vi "D3X86 GPIB Error check.vi"(1 "GPIB Error":i16, 2 "Status":bool[](array[boolean])) -> (0 "Error":bool)   [LabVIEW 2017]
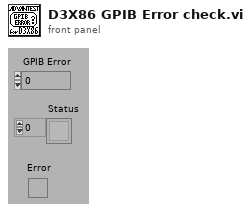
[diagram p1: front panel]
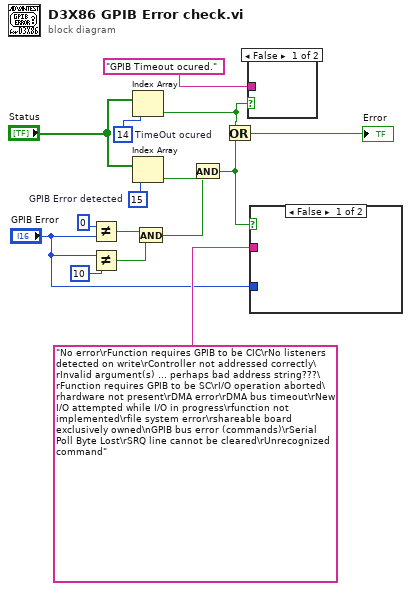
[diagram p0: block diagram]
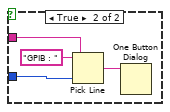
[diagram p2: hidden frame]
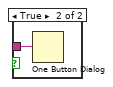
[diagram p3: hidden frame]
diagram:
  w14 = 14  # TimeOut ocured
  w15 = 15  # GPIB Error detected
  n1 = Not Equal?(x=u16 0, y="GPIB Error") -> (x != y?=w2:bool)
  n2 = Not Equal?(x="GPIB Error", y=10) -> (x != y?=w1:bool)
  n3 = Index Array(array="Status", index=w14) -> (element=w9:bool)
  n4 = Index Array(array="Status", index=w15) -> (element=w13:bool)
  n5 = And(x=w2, y=w1) -> (x .and. y?=w3:bool)
  n6 = And(x=w13, y=w3) -> (x .and. y?=w8:bool)
  n7 = Or(x=w9, y=w8) -> (x .or. y?=→"Error":bool)
  n8 = case shown="False" w9 {
    tunnel: "GPIB Timeout ocured." -> [_ w16]
    frame False {
    }
    frame True {
      n9 = One Button Dialog(message=w16) -> ()  [unwired: 1 in, 1 out]
    }
  }
  n10 = case shown="False" w8 {
    tunnel: "GPIB Error" -> [_ w19]
    tunnel: "No error\rFunction requires GPIB to be CIC\rNo listeners detected on write\rController not addressed correctly\rInvalid argument(s) ... perhaps bad address string???\rFunction requires GPIB to be SC\rI/O operation aborted\rhardware not present\rDMA error\rDMA bus timeout\rNew I/O attempted while I/O in progress\rfunction not implemented\rfile system error\rshareable board exclusively owned\nGPIB bus error (commands)\rSerial Poll Byte Lost\rSRQ line cannot be cleared\rUnrecognized command" -> [_ w18]
    frame False {
    }
    frame True {
      n11 = Pick Line(string ("")="GPIB : ", multi-line string=w18, line index=w19) -> (output string=w20:string)
      n12 = One Button Dialog(message=w20) -> ()  [unwired: 1 in, 1 out]
    }
  }
